vi "1LCR Meter Acquire Single_1.vi"() -> ()   [LabVIEW 2021, in "LCR Meter.lvlib"]
doc: "This example shows how to configure a measurement and take a reading."
uses:
  <vilib>/LCR Meter.lvlib
panel:
  out "Boolean":bool
  in  "stop":bool
  out "Monitor2 Value":dbl
  out "Monitor1 Value":dbl
  out "Secondary Value":dbl
  out "Primary Value":dbl
  in  "DC Bias Voltage (0)":dbl min=-2.5 max=2.5 step=0.01
  in  "DC Bias":bool caption="BIAS"
  in  "Current Level (1)":dbl=1.0 min=0.1 max=20.0 step=0.01
  in  "Voltage Level (1)":dbl=1.0 min=0.01 max=2.0 step=0.01
  in  "Level Mode":u16(ring) items=["Voltage", "Current"]
  in  "ALC (F: Disable)":bool
  in  "Frequery (1000)":dbl=1000.0 min=10.0 max=300000.0 step=0.01
  in  "Monitor2":i32(ring) items=["OFF", "Z", "D", "Q", "THR", "THD", "R", "X", "G", "B", "Y", "ABS", "PER", "VAC", "IAC"]
  in  "Monitor1":i32(ring) items=["OFF", "Z", "D", "Q", "THR", "THD", "R", "X", "G", "B", "Y", "ABS", "PER", "VAC", "IAC"]
  in  "Speed (0: SLOW)":i32(ring) items=["SLOW", "MED", "FAST"]
  in  "Average (0)":i32 min=0 max=256 step=1
  in  "Auto Range (1: ON)":i32(ring)=1 items=["OFF", "ON", "NOM"]
  in  "Range (0: 0)":i32(ring) items=["0", "1", "2", "3", "4", "5", "6", "7", "8", "MIN", "MAX"]
  in  "Auto LCZ (T: Enable)":bool=TRUE
  in  "Function (0: Cs-Rs)":i32(ring) items=["Cs-Rs", "Cs-D", "Cp-Rp", "Cp-D", "Lp-Rp", "Lp-Q", "Ls-Rs", "Ls-Q", "Rs-Q", "Rp-Q", "R-X", "DCR", "Z-thr", "Z-thd", "Z-D", "Z-Q"]
  in  "Serial Settings:Baud Rate":u32(ring)=115200 items=["9600"=9600, "38400"=38400, "57600"=57600, "115200"=115200]
  in  "VISA resource name":refnum<visa-resource-name>
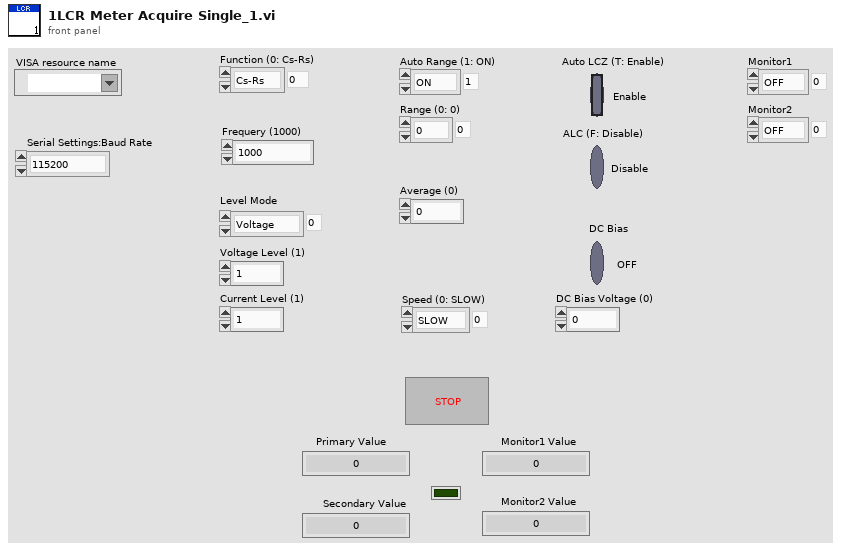
[diagram p1: front panel]
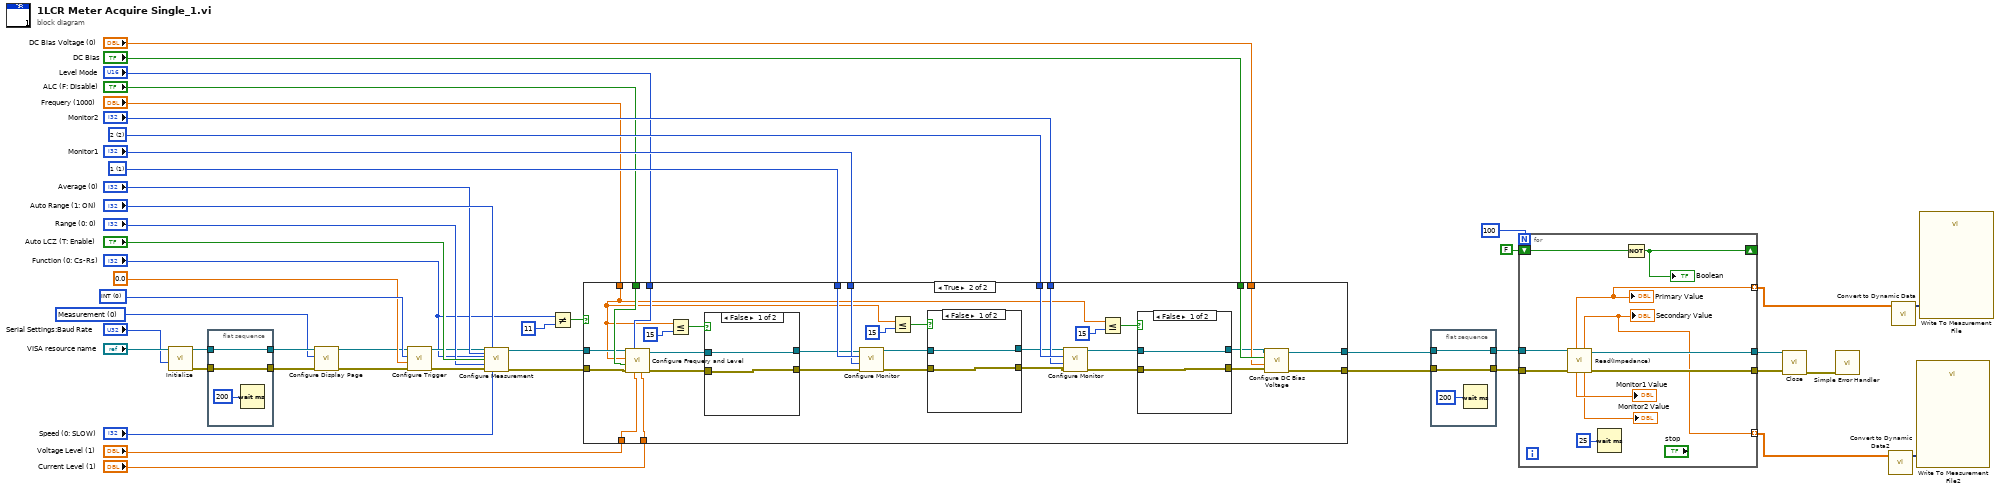
[diagram p0: block diagram]
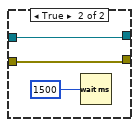
[diagram p3: hidden frame]
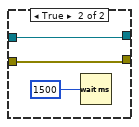
[diagram p4: hidden frame]
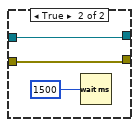
[diagram p5: hidden frame]
diagram:
  w14 = u16 0 items=["Measurement", "Measurement Setup", "BIN Measurement", "BIN Count", "BIN Setup", "LIST Measurement", "LIST Setup", "CORRECTION", "CATALOG", "ENLARGE", "System Config", "System Information"] ("Display Page")
  w26 = 0 items=["INT", "MAN", "EXT", "BUS"] ("Trigger Source (0: INT)")
  w36 = 2 items=["1"=1, "2"=2] ("Monitor (1)")
  w38 = 1 items=["1"=1, "2"=2] ("Monitor (1)")
  n1 = call <vilib>:"Initialize.vi"("Serial Settings:Baud Rate"="Serial Settings:Baud Rate", "VISA resource name"="VISA resource name") -> ("error out"=w17:errorcluster, "VISA resource name out"=w20:refnum<visa-resource-name>)  [unwired: 7 in, 1 out]
  n2 = flat-sequence {
    tunnel: [w50] -> w19
    tunnel: w20 -> [w50]
    tunnel: w17 -> [w49]
    tunnel: [w49] -> w16
    frame #0 {
      n3 = Wait (ms)(milliseconds to wait=u32 200) -> ()  [unwired: 1 out]
    }
  }
  n4 = call <vilib>:"Configure Display Page.vi"("error in"=w16, "Display Page"=w14, "VISA resource name"=w19) -> ("error out"=w15:errorcluster, "VISA resource name out"=w18:refnum<visa-resource-name>)  [unwired: 7 in]
  n5 = call <vilib>:"Configure Trigger.vi"("error in (no error)"=w15, "Trigger Delay (0)"=0.0, "Trigger Source (0: INT)"=w26, "VISA resource name"=w18) -> ("error out"=w27:errorcluster, "VISA resource name out"=w28:refnum<visa-resource-name>)  [unwired: 6 in]
  n6 = call <vilib>:"Configure Measurement.vi"("VISA resource name"=w28, "Auto Range (1: ON)"="Auto Range (1: ON)", "Average (0)"="Average (0)", "Function (0: Cs-Rs)"="Function (0: Cs-Rs)", "Auto LCZ (T: Enable)"="Auto LCZ (T: Enable)", "Range (0: 0)"="Range (0: 0)", "error in (no error)"=w27, "Speed (0: SLOW)"="Speed (0: SLOW)") -> ("VISA resource name out"=w40:refnum<visa-resource-name>, "error out"=w39:errorcluster)  [unwired: 6 in]
  n7 = Not Equal?(x="Function (0: Cs-Rs)", y=11) -> (x != y?=w13:bool)
  n8 = case shown="True" w13 {
    tunnel: w40 -> [w52 w73]
    tunnel: w39 -> [w51 w72]
    tunnel: w38 -> [_ w85]
    tunnel: "Monitor1" -> [_ w84]
    tunnel: w36 -> [_ w83]
    tunnel: "Monitor2" -> [_ w82]
    tunnel: "Frequery (1000)" -> [_ w53]
    tunnel: "ALC (F: Disable)" -> [_ w77]
    tunnel: "Level Mode" -> [_ w76]
    tunnel: "Voltage Level (1)" -> [_ w75]
    tunnel: "Current Level (1)" -> [_ w74]
    tunnel: "DC Bias" -> [_ w81]
    tunnel: "DC Bias Voltage (0)" -> [_ w80]
    tunnel: [w52 w79] -> w9
    tunnel: [w51 w78] -> w8
    frame False {
    }
    frame True {
      n9 = call <vilib>:"Configure Frequery and Level.vi"("Current Level (1)"=w74, "Voltage Level (1)"=w75, "Level Mode"=w76, "error in (no error)"=w72, "ALC (F: Disable)"=w77, "Frequery (1000)"=w53, "VISA resource name"=w73) -> ("error out"=w69:errorcluster, "VISA resource name out"=w68:refnum<visa-resource-name>)  [unwired: 3 in]
      n10 = Less Or Equal?(x=w53, y=15) -> (x <= y?=w70:bool)
      n11 = case shown="False" w70 {
        tunnel: w68 -> [w97 w99]
        tunnel: w69 -> [w96 w98]
        tunnel: [w97 w99] -> w66
        tunnel: [w96 w98] -> w67
        frame False {
        }
        frame True {
          n12 = Wait (ms)(milliseconds to wait=u32 1500) -> ()  [unwired: 1 out]
        }
      }
      n13 = call <vilib>:"Configure Monitor.vi"("error in (no error)"=w67, "Parameter (0: OFF)"=w84, "Monitor (1)"=w85, "VISA resource name"=w66) -> ("error out"=w58:errorcluster, "VISA resource name out"=w61:refnum<visa-resource-name>)  [unwired: 6 in]
      n14 = Less Or Equal?(x=w53, y=15) -> (x <= y?=w64:bool)
      n15 = case shown="False" w64 {
        tunnel: w61 -> [w92 w94]
        tunnel: w58 -> [w91 w93]
        tunnel: [w92 w94] -> w60
        tunnel: [w91 w93] -> w57
        frame False {
        }
        frame True {
          n16 = Wait (ms)(milliseconds to wait=u32 1500) -> ()  [unwired: 1 out]
        }
      }
      n17 = call <vilib>:"Configure Monitor.vi"("error in (no error)"=w57, "Parameter (0: OFF)"=w82, "Monitor (1)"=w83, "VISA resource name"=w60) -> ("error out"=w56:errorcluster, "VISA resource name out"=w59:refnum<visa-resource-name>)  [unwired: 6 in]
      n18 = Less Or Equal?(x=w53, y=15) -> (x <= y?=w62:bool)
      n19 = case shown="False" w62 {
        tunnel: w59 -> [w87 w89]
        tunnel: w56 -> [w86 w88]
        tunnel: [w87 w89] -> w55
        tunnel: [w86 w88] -> w54
        frame False {
        }
        frame True {
          n20 = Wait (ms)(milliseconds to wait=u32 1500) -> ()  [unwired: 1 out]
        }
      }
      n21 = call <vilib>:"Configure DC Bias Voltage.vi"("VISA resource name"=w55, "DC Bias"=w81, "DC Bias Voltage (0)"=w80, "error in (no error)"=w54) -> ("VISA resource name out"=w79:refnum<visa-resource-name>, "error out"=w78:errorcluster)  [unwired: 5 in]
    }
  }
  n22 = flat-sequence {
    tunnel: [w103] -> w7
    tunnel: w9 -> [w103]
    tunnel: w8 -> [w102]
    tunnel: [w102] -> w6
    frame #0 {
      n23 = Wait (ms)(milliseconds to wait=u32 200) -> ()  [unwired: 1 out]
    }
  }
  n24 = for {
    N: 100 -> [_]
    tunnel: w6 -> [w115]
    tunnel: [w110] -> w24
    tunnel: [w109] -> w23
    shift-right: [w107] -> _
    shift-left: FALSE -> [w108]
    tunnel: w7 -> [w106]
    tunnel: [w105] -> w4 mode=indexing
    tunnel: [w104] -> w2 mode=indexing
    n25 = call <vilib>:"Read(Impedance).vi"("error in (no error)"=w115, "VISA resource name"=w106) -> ("error out"=w109:errorcluster, "VISA resource name out"=w110:refnum<visa-resource-name>, "Monitor2 Value"=→"Monitor2 Value":dbl, "Secondary Value"=w104:dbl, "Monitor1 Value"=→"Monitor1 Value":dbl, "Primary Value"=w105:dbl)  [unwired: 3 in, 1 out]
    "Primary Value" <- w105
    "Secondary Value" <- w104
    n26 = Wait (ms)(milliseconds to wait=u32 25) -> ()  [unwired: 1 out]
    n27 = Not(x=w108) -> (.not. x?=w107:bool)
    "Boolean" <- w107
  }
  n28 = call <vilib>:"Close.vi"("error in (no error)"=w23, "VISA resource name"=w24) -> ("error out"=w22:errorcluster)  [unwired: 9 in]
  n29 = call <vilib>:"Simple Error Handler.vi"("error in (no error)"=w22) -> ()  [unwired: 4 in, 5 out]
  n30 = call "Convert to Dynamic Data2"("Array"=w2) -> ("Dynamic Data Type"=w1:dynamicdata)  [unwired: 3 in]
  n31 = call "Convert to Dynamic Data"("Array"=w4) -> ("Dynamic Data Type"=w3:dynamicdata)  [unwired: 3 in]
  n32 = call "Write To Measurement File2"("Signals"=w1) -> ()  [unwired: 16 in, 3 out]
  n33 = call "Write To Measurement File"("Signals"=w3) -> ()  [unwired: 16 in, 3 out]
